vi "Data averaging.vi"(3 "data":dbl[][](array[numeric]) format="%0.2f") -> (1 "Averaged data":dbl[][](array[numeric]))   [LabVIEW 2012]
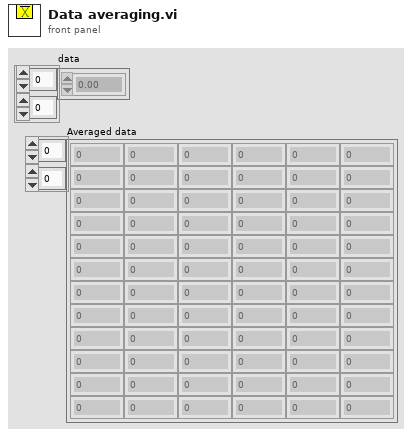
[diagram p1: front panel]
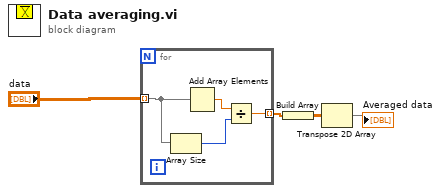
[diagram p0: block diagram]
diagram:
  n1 = for {
    tunnel: "data" -> [w8] mode=indexing
    tunnel: [w5] -> w4 mode=indexing
    n2 = Array Size(array=w8) -> (size(s)=w6:i32)
    n3 = Add Array Elements(numeric array=w8) -> (sum=w7:dbl)
    n4 = Divide(x=w7, y=w6) -> (x/y=w5:dbl)
  }
  n5 = Build Array(w4) -> (w3:dbl[][])
  n6 = Transpose 2D Array(2D array=w3) -> (transposed array=→"Averaged data":dbl[][])
